vi "Initialize Waypoint List.vi"(11 "GPS Waypoint CSV Path":path) -> (3 "Waypoint Array":T1(array[cluster]))   [LabVIEW 2011]
uses:
  <vilib>/Utility/file.llb/Read From Spreadsheet File (DBL).vi
panel:
  in  "GPS Data 2":T2 {"Time"."GPS Time of Week" format="%.3f"; "Velocity, Correction & SET"."Extended Navigation Mode" items=["Non Differential"=0, "Code (RTCM Type 1 & 9)"=1, "Code, Single Frequency (WAAS)"=2, "Code, Dual Frequency (WAAS)"=3, "Code, Single Frequency (WCT)"=4, "Code/RCP, Dual Frequency (WCT)"=5, "Code, Single Frequency (RTG)"=6, "Code (RTCM Type 1 & 9) Dual Frequency"=10, "Code/RCP, Dual Frequency (RTG)"=11, "Code, Single Frequency (NCT-RTK)"=12, "Code, Single Frequency (RTCM 18 & 19)"=13, "Code, Single Frequency (RTCM 21 & 22)"=14, "Code, Single Frequency (CMR)"=15, "Code, Dual Frequency (NCT-RTK)"=16, "Code, Dual Frequency (RTCM 18 & 19)"=17, "Code, Dual Frequency (RTCM 20 & 21)"=18, "Code, Dual Frequency (CMR)"=19, "RTK (NCT-RTK)"=20, "RTK (RTCM 18 & 19)"=21, "RTK (RTCM 20 & 21)"=22, "RTK (CMR)"=23, "Code, Single Frequency with SET (RTG)"=24, "Code/RCP, Dual Frequency with SET (RTG)"=25, "RTK Extend"=26]}
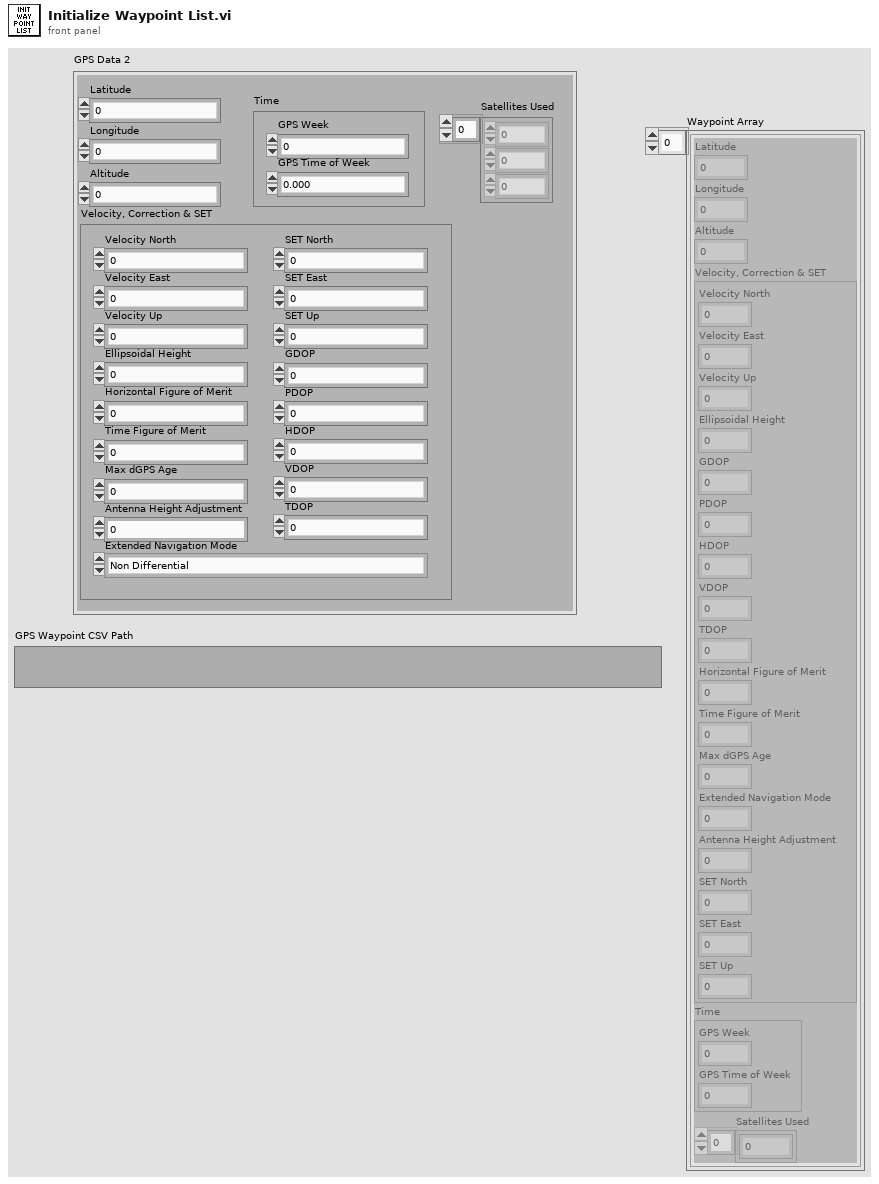
[diagram p1: front panel]
types:
  T1 = cluster{"Latitude":dbl, "Longitude":dbl, "Altitude":dbl, "Velocity, Correction & SET":cluster{"Velocity North":dbl, "Velocity East":dbl, "Velocity Up":dbl, "Ellipsoidal Height":dbl, "GDOP":sgl, "PDOP":sgl, "HDOP":sgl, "VDOP":sgl, "TDOP":sgl, "Horizontal Figure of Merit":u8, "Time Figure of Merit":u8, "Max dGPS Age":sgl, "Extended Navigation Mode":u8, "Antenna Height Adjustment ":dbl, "SET North":i32, "SET East":i32, "SET Up":i32}, "Time":cluster{"GPS Week":u16, "GPS Time of Week":sgl}, "Satellites Used":i32[]}[]
  T2 = cluster{"Latitude":dbl, "Longitude":dbl, "Altitude":dbl, "Velocity, Correction & SET":cluster{"Velocity North":dbl, "Velocity East":dbl, "Velocity Up":dbl, "Ellipsoidal Height":dbl, "GDOP":sgl, "PDOP":sgl, "HDOP":sgl, "VDOP":sgl, "TDOP":sgl, "Horizontal Figure of Merit":u8, "Time Figure of Merit":u8, "Max dGPS Age":sgl, "Extended Navigation Mode":u8, "Antenna Height Adjustment ":dbl, "SET North":i32, "SET East":i32, "SET Up":i32}, "Time":cluster{"GPS Week":u16, "GPS Time of Week":sgl}, "Satellites Used":i32[]}
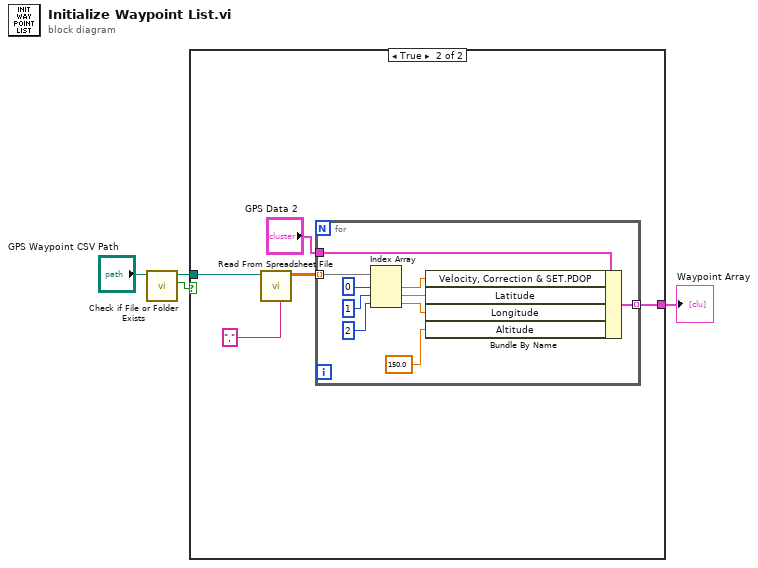
[diagram p0: block diagram]
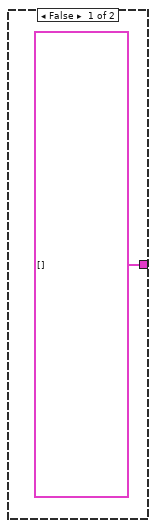
[diagram p2: hidden frame]
diagram:
  n1 = call <vilib>:"Check if File or Folder Exists.vi"("path"="GPS Waypoint CSV Path") -> ("file or folder exists?"=w1:bool, "dup path"=w2:path)  [unwired: 8 in, 1 out]
  n2 = case shown="True" w1 {
    tunnel: [T1 [] w7] -> w4
    tunnel: w2 -> [_ w6]
    frame False {
    }
    frame True {
      n3 = call-poly <vilib>:"Read From Spreadsheet File.vi"("delimiter (\\t)"="," ("delimiter (\\t)"), "file path (dialog if empty)"=w6) -> ("all rows"=w9:dbl[][])  [unwired: 5 in, 4 out]
      n4 = for {
        tunnel: w9 -> [w16] mode=indexing
        tunnel: "GPS Data 2" -> [w20]
        tunnel: [w12] -> w7 mode=indexing
        n5 = Index Array(array=w16, index #1=0 ("index"), index #2=1 ("index"), index #3=2 ("index")) -> (element #1=w11:dbl, element #2=w15:dbl, element #3=w14:dbl)
        n6 = Bundle By Name(cluster=w20, "Velocity, Correction & SET.PDOP"=w11, "Latitude"=w15, "Longitude"=w14, "Altitude"=150.0) -> (w12:T2)
      }
    }
  }
  "Waypoint Array" <- w4
